vi "REC TRACE.vi"(0 "System no.":i32=1 min=1 max=4 step=1, 2 "List of Data Recorder Trace Configurations":T1[](array[typedef]) {"ParameterID" min=1 max=4 step=1 format="%x"; "TraceID" min=1 max=4 step=1}, 5 "error in":errorcluster) -> (19 "error out":errorcluster)   [LabVIEW 2020]
doc: "REC TRACE (Configure Data Recorder Trace)\n\nDescription\nConfigures a trace of a data recorder for recording:\nAssigns the variable to be recorded to the trace. The variable must be a parameter. The \npermitted parameter types can be queried with USG? PROP (p. 79). \nA data recorder can only be configured when it is in the state \"CFG\", see the state diagram for \nthe data recorder (p. 110). The state of the data recorder can be queried with REC? STATE\n(p. 47). \n\nFormat\nREC TRACE <RecorderID> <TraceID> <Container Unit> <Function Unit> <ParameterID>\n\nArguments\n<RecorderID>\nData recorder, whose trace is to be configured; to be specified as alias (p. 94) \nThe available data recorders can be queried with USG? SYS (p. 80). \nPossible values: REC_1 to RECn, where n = number of data recorders in the controller\n<TraceID>\nID of the trace to be configured\nThe number of traces of the data recorder can be queried via parameter 0x104. Example:\n>>spv? ram rec_1 - 0x104\n<<RAM REC_1 - 0x104=4\nPossible values: 1 to n, where n = Number of traces of the data recorder\n<Container Unit>\nContainer unit, whose parameter is to be recorded\nThe existing container units can be queried with USG? SYS.\nPossible values: Alias of the container unit (p. 94) \n<Function Unit>\nFunction unit, whose parameter is to be recorded \nThe existing function units can be queried with USG? SYS.\nIf a parameter belonging to a container unit is to be recorded, \"-\" must be entered for \n<Function Unit>.\nPossible values:\nAlias of the function unit (p. 94) \n\"-\" \n<ParameterID>\n<ParameterID> specifies the variable to be recorded (permitted parameter types can be queried \nwith USG? PROP).\n<ParameterID> always contains a parameter identifier in hexadecimal format. For 0-\ndimensional parameters, <ParameterID> is fully specified by the parameter identifier.\nFor one-dimensional and multi-dimensional parameters, an element address is also required \ntogether with the parameter identifier. Depending on the dimension of the parameter, the \nelement address consists of one or more parts that are separated from the parameter identifier \nand each other by a comma.\n- One-dimensional parameter (vector) ? the element address is ,number\n- Two-dimensional parameter (two-dimensional matrix) ? the element address is \n,number,number\n- Three-dimensional parameter (three-dimensional matrix) ? the element address \nis ,number,number,number\nThe address data for the parameters can be queried with USG? PAM (p. 77). \nPossible values:\n0x0000 to 0xFFFF\nFor one-dimensional and multi-dimensional parameters, an additional integer = 1 for each \ndimension\n\nResponse\nnone\n\nExample\nIn trace 1, data recorder 1 is to record the target position for the first axis of the controller. The \ntarget position belongs directly to container unit Axis_1 as parameter 0x101 (see the response \nto USG? PAM (p. 77)).\n>>rec trace rec_1 1 axis_1 - 0x101\nIn trace 2, data recorder 1 is to record the controller output for the first controller of the first \naxis (parameter 0x103, see response to USG? PAM).\n>>rec trace rec_1 2 axis_1 cntr_1 0x103\nIn trace 3, data recorder 2 is to record the first element of the vector \"Position Sensor\" for the \ncontainer unit CON_1 (parameter 0x102, see the response to USG? PAM), and the second \nelement of this vector in trace 4.\n>>rec trace rec_2 3 con_1 - 0x102,1\n>>rec trace rec_2 4 con_1 - 0x102,2\n\nNotes\nThe number of available traces and points per trace depends on the memory management in \nthe controller.\nIf one or more traces of the data recorder are configured, the data stored in all traces of this \ndata recorder will be deleted.\nFor further details, see \"Data Recorder - GCS 3.0\" (p. 107). \n\nUser command level\nUSR"
uses:
  RecorderTraceConfiguration.ctl
panel:
  # "REC TRACE (Configure Data Recorder Trace)\n\nConfigures a trace of a data recorder for recording:\nAssigns the variable to be recorded to the trace. The variable must be a parameter. The \npermitted parameter types can be queried with USG? PROP. \nA data recorder can only be configured when it is in the state \"CFG\", see the state diagram for the data recorder. The state of the data recorder can be queried with REC? STATE."
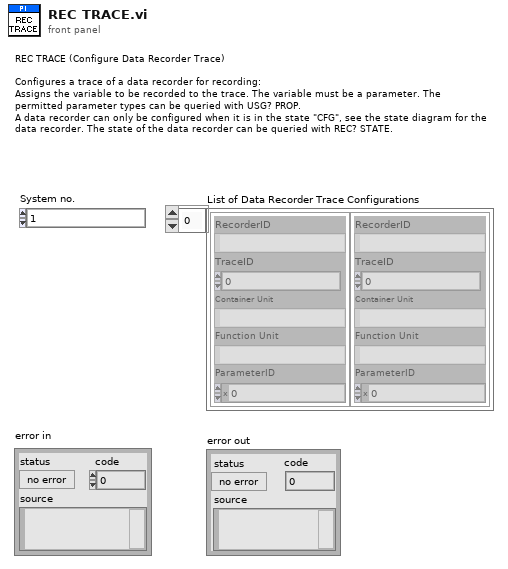
[diagram p1: front panel]
types:
  T1 = typedef "RecorderTraceConfiguration.ctl" = cluster{"RecorderID":string, "TraceID":i32, "Container Unit":string, "Function Unit":string, "ParameterID":i32}
  T2 = typedef "Syntax.ctl" = enum16{"GCS 1.0", "GCS 2.0", "GCS 3.0"}
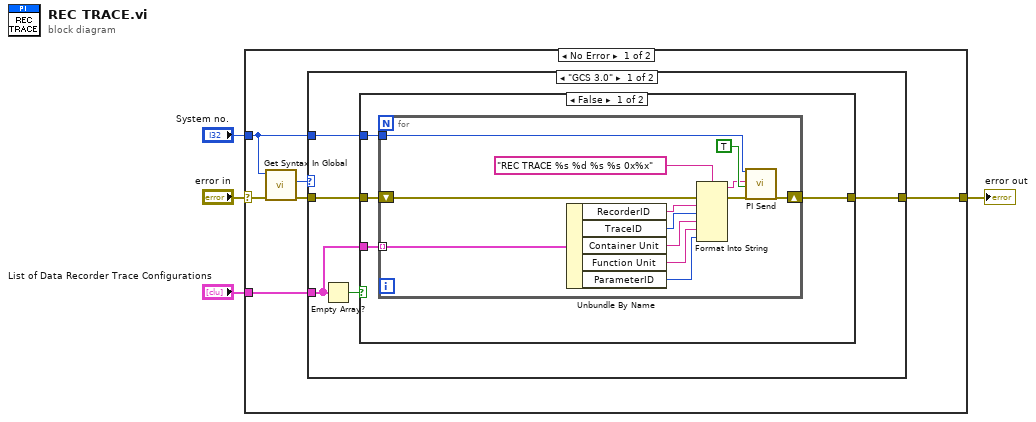
[diagram p0: block diagram]
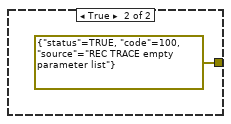
[diagram p2: hidden frame]
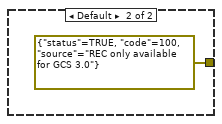
[diagram p3: hidden frame]
diagram:
  n1 = case shown="No Error" "error in" {
    selector: "error in" -> [w10 w35]
    tunnel: [w7 w35] -> w2
    tunnel: "System no." -> [w6 _]
    tunnel: "List of Data Recorder Trace Configurations" -> [w5 _]
    frame No Error {
      n2 = call "Get Syntax In Global.vi"("error in"=w10, "System no."=w6) -> ("error out"=w8:errorcluster, "Syntax"=w9:T2)  [unwired: 8 in]
      n3 = case shown="\"GCS 3.0\"" w9 {
        tunnel: w8 -> [w15 _]
        tunnel: [w14 errorcluster {"status"=TRUE, "code"=100, "source"="REC only available for GCS 3.0"} ("error out")] -> w7
        tunnel: w6 -> [w13 _]
        tunnel: w5 -> [w11 _]
        frame "GCS 3.0" {
          n4 = Empty Array?(array=w11) -> (empty?=w12:bool)
          n5 = case shown="False" w12 {
            tunnel: w15 -> [w19 _]
            tunnel: [w18 errorcluster {"status"=TRUE, "code"=100, "source"="REC TRACE empty parameter list"} ("error out")] -> w14
            tunnel: w13 -> [w17 _]
            tunnel: w11 -> [w16 _]
            frame False {
              n6 = for {
                shift-right: [w29] -> w18
                shift-left: w19 -> [w31]
                tunnel: w17 -> [w26]
                tunnel: w16 -> [w25] mode=indexing
                n7 = Unbundle By Name(w25) -> ("RecorderID"=w24:string, "TraceID"=w23:i32, "Container Unit"=w22:string, "Function Unit"=w21:string, "ParameterID"=w20:i32)
                n8 = Format Into String(format string="REC TRACE %s %d %s %s 0x%x", error in=w31, w24, w23, w22, w21, w20) -> (resulting string=w27:string, error out=w30:errorcluster)  [unwired: 1 in]
                n9 = call "PI Send.vi"("System no."=w26, "String to send"=w27, "Attach termination char.?"=TRUE, "error in"=w30) -> ("error out"=w29:errorcluster)  [unwired: 2 in, 13 out]
              }
            }
            frame True {
            }
          }
        }
        frame Default {
        }
      }
    }
    frame Error {
    }
  }
  "error out" <- w2
